vi "SampleListWindow.vi"() -> ()   [LabVIEW 2013]
doc: "The UI for the SampleList that handles the processing of multile samples"
uses:
  Classes/Flags/flag.lvclass
panel:
  out "Analysis Clipboard":string[](array[string])
  out "next sample":u16
  in  "Save button":bool
  in  "load button":bool
  in  "Add sample button":bool
  in  "Add blank button":bool
  out "error out":errorcluster
  in  "error in (no error)":errorcluster
  in  "Start/Stop Button":bool
  in  "Delete Button":bool
  in  "Add std button":bool
  in  "SampleList":i32(listbox)
  # "Add to list"
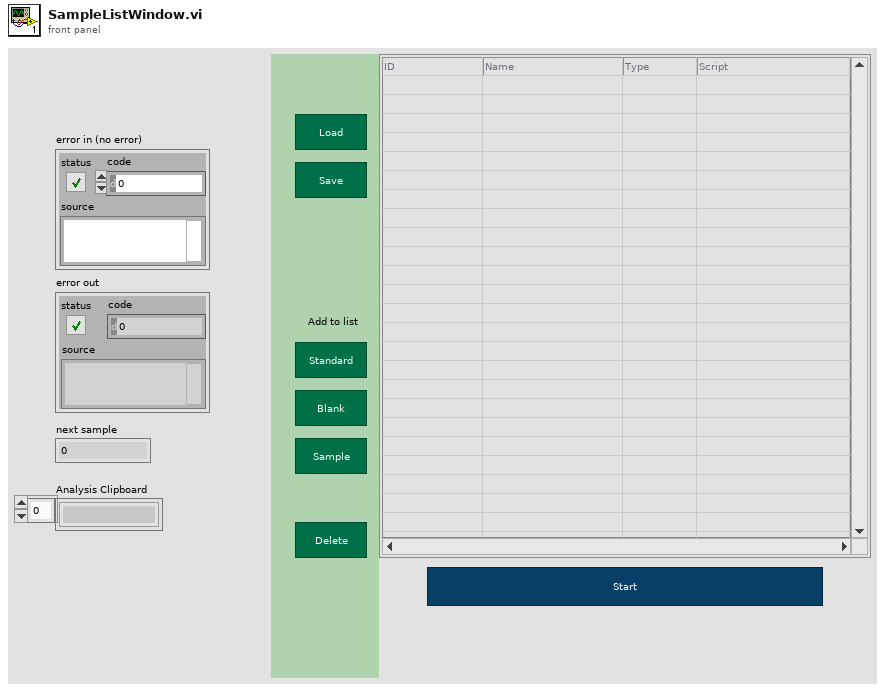
[diagram p1: front panel]
types:
  T1 = typedef "eventvkey.ctl" = enum16{"ASCII", "Enter", "Return", "Shift", "Ctrl", "Alt", "Cmd", "Opt", "Caps", "NumLock", "Clear", "Break", "Up", "Down", "Left", "Right", "Insert", "Delete", "Home", "End", "PageUp", "PageDown", "Escape", "Help", "Pause", "ScrollLock", "F1", "F2", "F3", "F4", "F5", "F6", "F7", "F8", "F9", "F10", "F11", "F12", "F13", "F14", "F15", "F16", "F17", "F18", "F19", "F20", "F21", "F22", "F23", "F24", "Play", "VolumeUp", "VolumeDown", "Mute", "Two Byte Char"}
  T2 = cluster{"Shift":bool, "Ctrl":bool, "Alt":bool, "Cmd":bool, "Opt":bool}
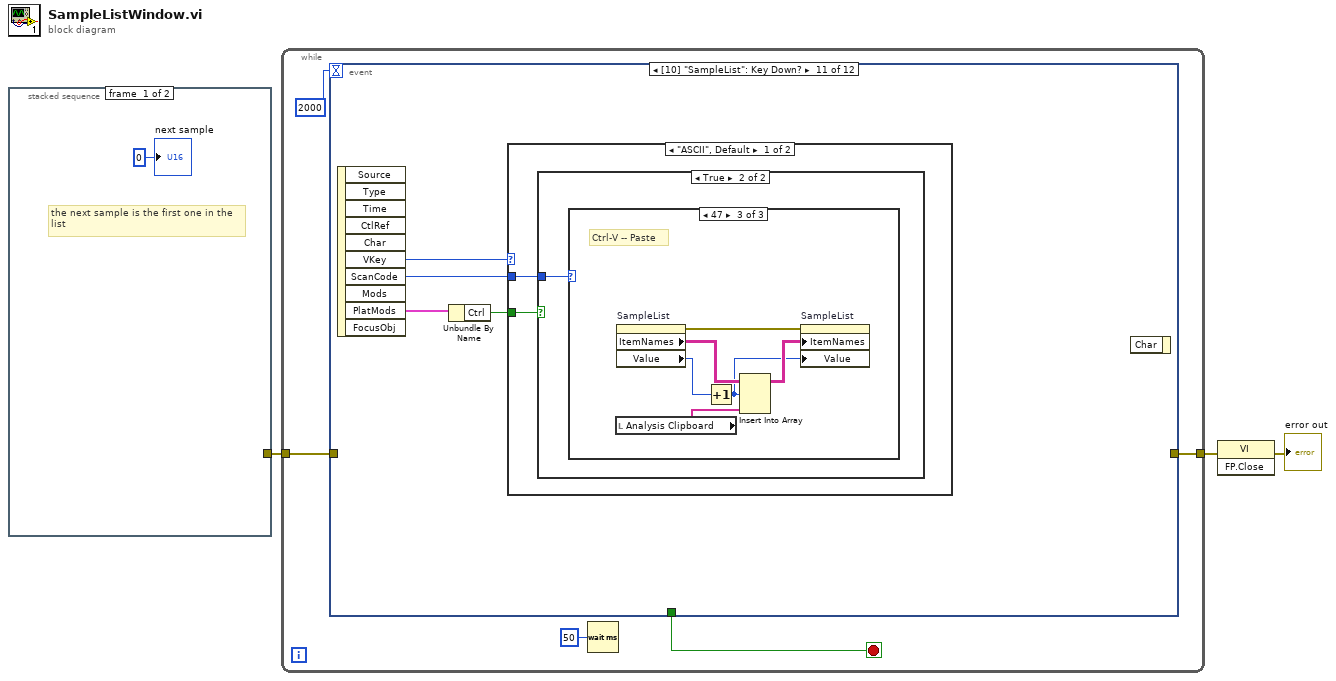
[diagram p0: block diagram]
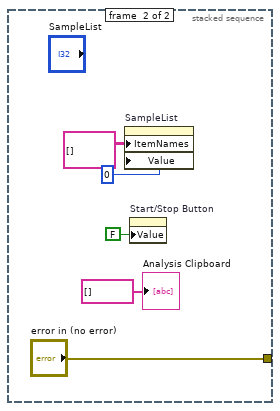
[diagram p2: hidden frame]
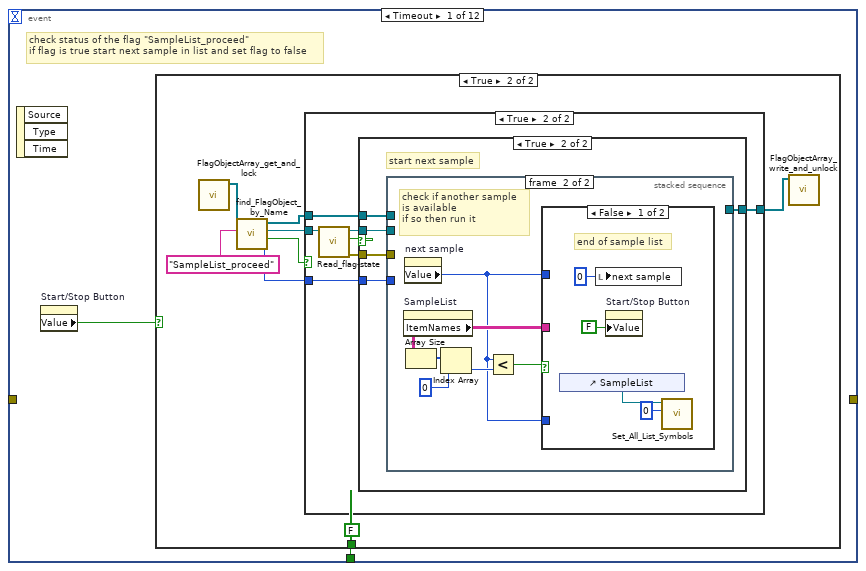
[diagram p3: hidden frame]
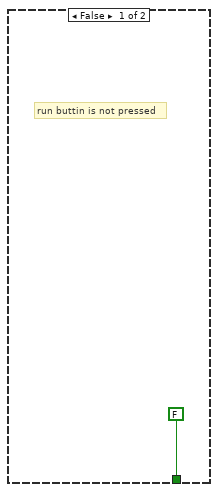
[diagram p4: hidden frame]
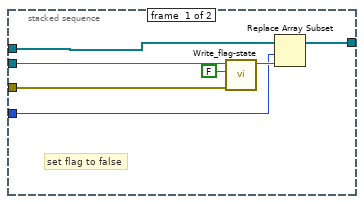
[diagram p7: hidden frame]
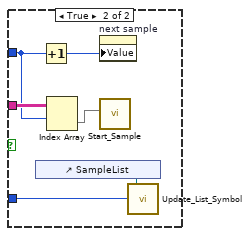
[diagram p8: hidden frame]
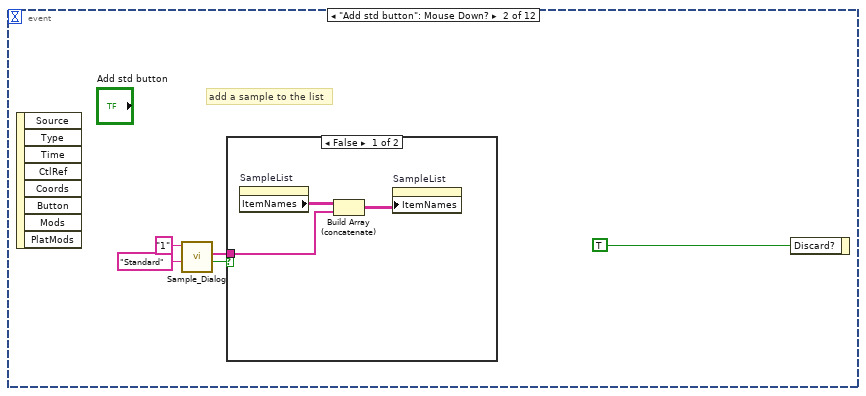
[diagram p9: hidden frame]
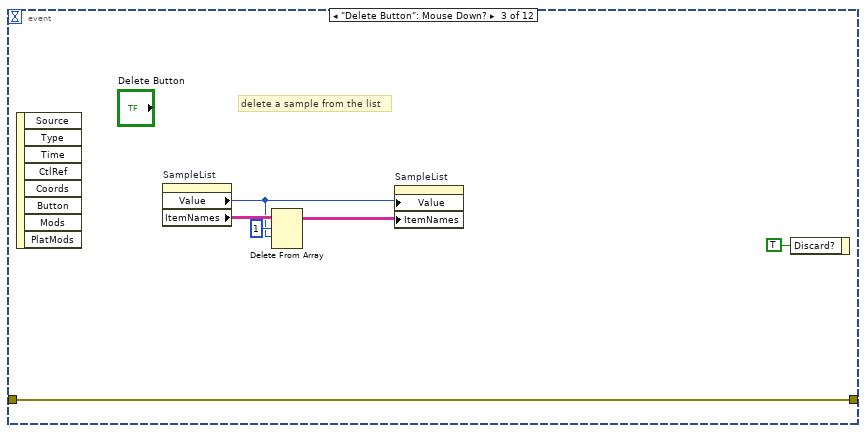
[diagram p11: hidden frame]
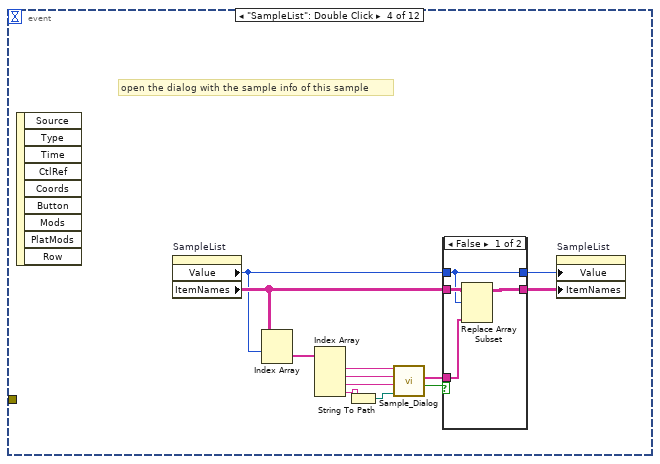
[diagram p12: hidden frame]
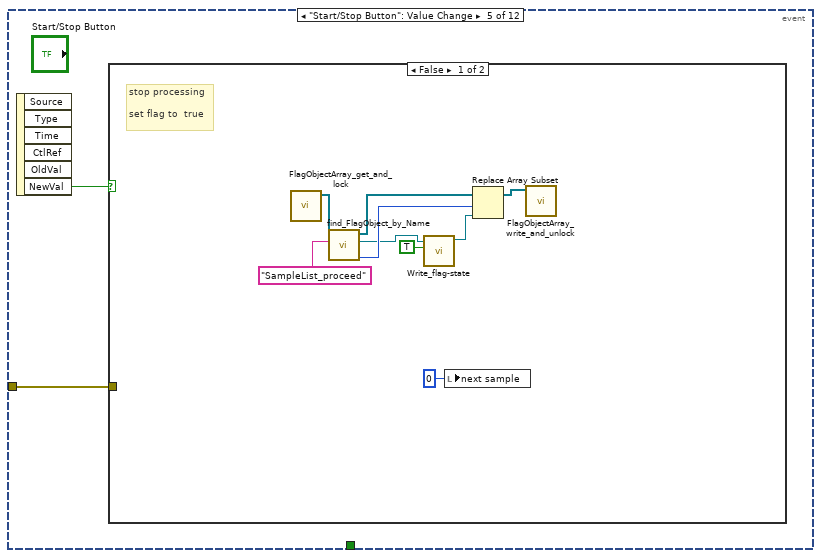
[diagram p14: hidden frame]
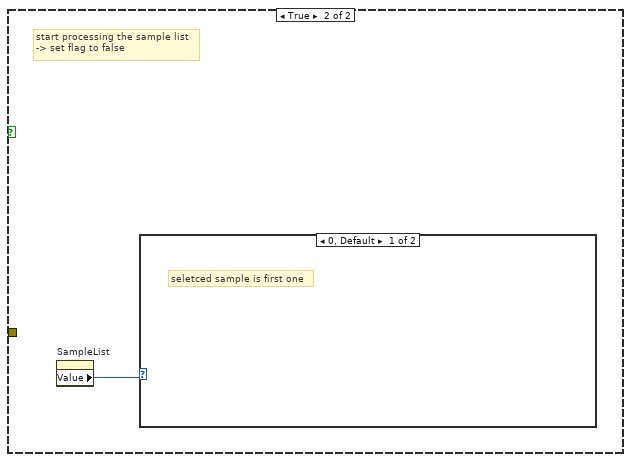
[diagram p15: hidden frame]
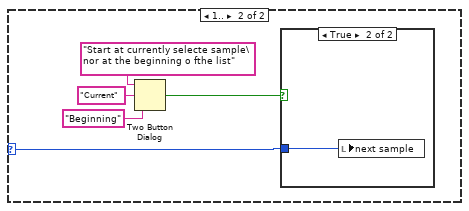
[diagram p16: hidden frame]
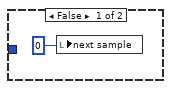
[diagram p17: hidden frame]
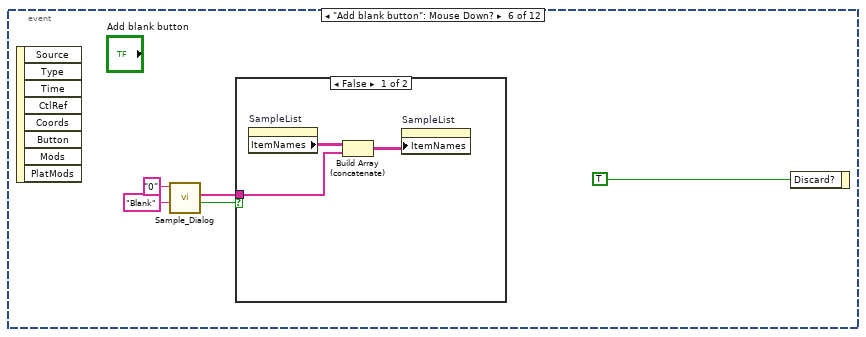
[diagram p18: hidden frame]
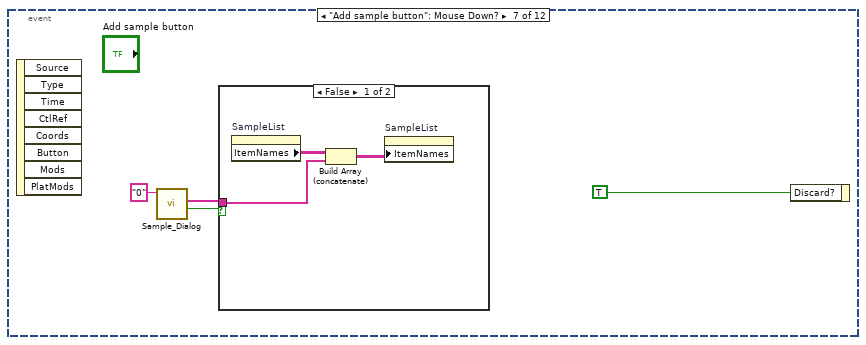
[diagram p20: hidden frame]
diagram:
  n1 = stacked-sequence {
    tunnel: [_ "error in (no error)"] -> w3
    frame #0 {
      # "the next sample is the first one in the\nlist"
      "next sample" <- u16 0 ("current sample")
    }
    frame #1 {
      n2 = property on="SampleList" class="MCListbox (strict)"("ItemNames"=string[][] [] ("Item Names"), "Value"=0 ("SampleList")) -> ()  [unwired: 2 in, 2 out]
      n3 = property on="Start/Stop Button" class="Bool (strict)"("Value"=FALSE ("Start/Stop Button")) -> ()  [unwired: 2 in, 2 out]
      "Analysis Clipboard" <- string[] [] ("Analysis Clipboard")
    }
  }
  n4 = while {
    tunnel: w3 -> [w12]
    tunnel: [w11] -> w2
    stop <- w14 stop-if-true
    n5 = event shown="[10] \"SampleList\": Key Down?" {
      selector: _ -> [_ _ _ _ _ _ _ _ _ _ _ _]
      dyn-events: _ -> [_ _ _ _ _ _ _ _ _ _ _ _]
      timeout: 2000 -> [_ _ _ _ _ _ _ _ _ _ _ _]
      tunnel: [w16 _ _ _ _ _ _ _ _ _ _ w193] -> w14
      tunnel: w12 -> [_ _ w76 _ w96 _ _ _ _ _ _ w191]
      tunnel: [_ _ w76 _ _ _ _ _ _ _ _ w191] -> w11
      event Timeout {
        # "check status of the flag \"SampleList_proceed\"\nif flag is true start next sample in list and set flag to false"
        n6 = event-data() -> ()  [unwired: 1 in, 3 out]
        n7 = property on="Start/Stop Button" class="Bool (strict)"() -> ("Value"=w15:bool)  [unwired: 2 in, 2 out]
        n8 = case shown="True" w15 {
          tunnel: [FALSE FALSE] -> w16
          frame False {
            # "run buttin is not pressed"
          }
          frame True {
            n9 = call "FlagObjectArray_get_and_lock.vi"() -> ("FlagObjects"=w24:refnum<class "flag.lvclass">[])  [unwired: 10 in, 1 out]
            n10 = call "find_FlagObject_by_Name.vi"("Flag Name"="SampleList_proceed", "FlagObj Array"=w24) -> ("index of Object in Array"=w18:i32, "found?"=w21:bool, "found FlagObj out"=w22:refnum<class "flag.lvclass">, "FlagObj Array out"=w20:refnum<class "flag.lvclass">[])  [unwired: 6 in]
            n11 = case shown="True" w21 {
              tunnel: w22 -> [_ w33]
              tunnel: w20 -> [w26 w31]
              tunnel: [w26 w29] -> w19
              tunnel: w18 -> [_ w27]
              frame False {
              }
              frame True {
                n12 = call-dynamic "Read_flag-state.vi"("flag in"=w33) -> ("error out"=w28:errorcluster, "flag state"=w30:bool, "flag out"=w32:refnum<class "flag.lvclass">)  [unwired: 8 in]
                n13 = case shown="True" w30 {
                  tunnel: w32 -> [_ w39]
                  tunnel: w31 -> [w34 w37]
                  tunnel: [w34 w35] -> w29
                  tunnel: w28 -> [_ w38]
                  tunnel: w27 -> [_ w36]
                  frame False {
                    # "do nothing, flag is still false"
                  }
                  frame True {
                    # "start next sample"
                    n14 = stacked-sequence {
                      tunnel: w39 -> [w46 _]
                      tunnel: w38 -> [w45 _]
                      tunnel: w37 -> [w43 _]
                      tunnel: w36 -> [w41 _]
                      tunnel: [w40 _] -> w35
                      frame #0 {
                        # "set flag to false"
                        n15 = call-dynamic "Write_flag-state.vi"("error in (no error)"=w45, "flag state"=FALSE, "flag in"=w46) -> ("flag out"=w42:refnum<class "flag.lvclass">)  [unwired: 7 in, 1 out]
                        n16 = Replace Array Subset(array=w43, new element=w42, index=w41) -> (w40:refnum<class "flag.lvclass">[])
                      }
                      frame #1 {
                        # "check if another sample\nis available\nif so then run it"
                        n17 = property on="SampleList" class="MCListbox (strict)"() -> ("ItemNames"=w52:string[][])  [unwired: 2 in, 2 out]
                        n18 = property on="next sample" class="DigNum (strict)"() -> ("Value"=w47:u16)  [unwired: 2 in, 2 out]
                        n19 = Array Size(array=w52) -> (size(s)=w51:i32[])
                        n20 = Index Array(array=w51, index=0) -> (element=w49:i32)
                        n21 = Less?(x=w47, y=w49) -> (x < y?=w48:bool)
                        n22 = case shown="False" w48 {
                          tunnel: w52 -> [_ w60]
                          tunnel: w47 -> [_ w59]
                          tunnel: w47 -> [_ w57]
                          frame False {
                            # "end of sample list"
                            n23 = control-ref of="SampleList"() -> (w54:refnum<vi>)
                            n24 = local write "next sample"(u16 0 ("next sample")) -> ()
                            n25 = property on="Start/Stop Button" class="Bool (strict)"("Value"=FALSE ("Start/Stop Button")) -> ()  [unwired: 2 in, 2 out]
                            n26 = call "Set_All_List_Symbols.vi"("symbol value"=u16 0, "MulticolumnListbox in"=w54) -> ()  [unwired: 10 in]
                          }
                          frame True {
                            n27 = control-ref of="SampleList"() -> (w58:refnum<vi>)
                            n28 = Increment(x=w59) -> (x+1=w61:u16)
                            n29 = Index Array(array=w60, index (row)=w59) -> (element=w62:string[])  [unwired: 1 in]
                            n30 = property on="next sample" class="DigNum (strict)"("Value"=w61) -> ()  [unwired: 2 in, 2 out]
                            n31 = call "Start_Sample.vi"("SampleList Data"=w62) -> ()  [unwired: 10 in, 1 out]
                            n32 = call "Update_List_Symbol.vi"("current sample"=w57, "MulticolumnListbox in"=w58) -> ()  [unwired: 10 in]
                          }
                        }
                      }
                    }
                  }
                }
              }
            }
            n33 = call "FlagObjectArray_write_and_unlock.vi"("FlagObjects"=w19) -> ()  [unwired: 10 in, 1 out]
          }
        }
      }
      event "Add std button": Mouse Down? {
        # "add a sample to the list"
        n34 = event-data() -> ()  [unwired: 1 in, 8 out]
        n35 = call "Sample_Dialog.vi"("Type"="Standard", "ID"="1") -> ("Canceled?"=w63:bool, "AnalysisData Out"=w64:string[])  [unwired: 8 in]
        n36 = case shown="False" w63 {
          tunnel: w64 -> [w68 _]
          frame False {
            n37 = property on="SampleList" class="MCListbox (strict)"() -> ("ItemNames"=w70:string[][])  [unwired: 2 in, 2 out]
            n38 = Build Array (concatenate)(w70, w68) -> (w69:string[][])
            n39 = property on="SampleList" class="MCListbox (strict)"("ItemNames"=w69) -> ()  [unwired: 2 in, 2 out]
          }
          frame True {
          }
        }
        n40 = event-data("Discard?"=TRUE) -> ()  [unwired: 1 in, 1 out]
      }
      event "Delete Button": Mouse Down? {
        # "delete a sample from the list"
        n41 = event-data() -> ()  [unwired: 1 in, 8 out]
        n42 = property on="SampleList" class="MCListbox (strict)"() -> ("Value"=w73:i32, "ItemNames"=w75:string[][])  [unwired: 2 in, 2 out]
        n43 = Delete From Array(array=w75, length=1, index (row)=w73) -> (array with subset deleted=w72:string[][])  [unwired: 1 in, 1 out]
        n44 = property on="SampleList" class="MCListbox (strict)"("Value"=w73, "ItemNames"=w72) -> ()  [unwired: 2 in, 2 out]
        n45 = event-data("Discard?"=TRUE) -> ()  [unwired: 1 in, 1 out]
      }
      event "SampleList": Double Click {
        # "open the dialog with the sample info of this sample"
        n46 = event-data() -> ()  [unwired: 1 in, 9 out]
        n47 = property on="SampleList" class="MCListbox (strict)"() -> ("Value"=w80:i32, "ItemNames"=w81:string[][])  [unwired: 2 in, 2 out]
        n48 = Index Array(array=w81, index (row)=w80) -> (element=w88:string[])  [unwired: 1 in]
        n49 = Index Array(array=w88) -> (element #1=w87:string, element #2=w86:string, element #3=w85:string, element #4=w84:string)  [unwired: 4 in]
        n50 = String To Path(string=w84) -> (path=w83:path)
        n51 = call "Sample_Dialog.vi"("Script"=w83, "Type"=w85, "Name"=w86, "ID"=w87) -> ("Canceled?"=w78:bool, "AnalysisData Out"=w79:string[])  [unwired: 6 in]
        n52 = case shown="False" w78 {
          tunnel: [w92 w94] -> w82
          tunnel: w81 -> [w91 w94]
          tunnel: w80 -> [w89 w93]
          tunnel: w79 -> [w90 _]
          tunnel: [w89 w93] -> w77
          frame False {
            n53 = Replace Array Subset(array=w91, new element=w90, index (row)=w89) -> (w92:string[][])  [unwired: 1 in]
          }
          frame True {
          }
        }
        n54 = property on="SampleList" class="MCListbox (strict)"("Value"=w77, "ItemNames"=w82) -> ()  [unwired: 2 in, 2 out]
      }
      event "Start/Stop Button": Value Change {
        n55 = event-data() -> ("NewVal"=w95:bool)  [unwired: 1 in, 5 out]
        n56 = case shown="False" w95 {
          tunnel: w96 -> [_ _]
          frame False {
            # "stop processing\n\nset flag to  true"
            n57 = call "FlagObjectArray_get_and_lock.vi"() -> ("FlagObjects"=w105:refnum<class "flag.lvclass">[])  [unwired: 10 in, 1 out]
            n58 = call "find_FlagObject_by_Name.vi"("Flag Name"="SampleList_proceed", "FlagObj Array"=w105) -> ("index of Object in Array"=w99:i32, "found FlagObj out"=w98:refnum<class "flag.lvclass">, "FlagObj Array out"=w100:refnum<class "flag.lvclass">[])  [unwired: 6 in, 1 out]
            n59 = call-dynamic "Write_flag-state.vi"("flag state"=TRUE, "flag in"=w98) -> ("flag out"=w102:refnum<class "flag.lvclass">)  [unwired: 8 in, 1 out]
            n60 = local write "next sample"(u16 0 ("next sample")) -> ()
            n61 = Replace Array Subset(array=w100, new element=w102, index=w99) -> (w101:refnum<class "flag.lvclass">[])
            n62 = call "FlagObjectArray_write_and_unlock.vi"("FlagObjects"=w101) -> ()  [unwired: 10 in, 1 out]
          }
          frame True {
            # "start processing the sample list\n-> set flag to false"
            n63 = property on="SampleList" class="MCListbox (strict)"() -> ("Value"=w106:i32)  [unwired: 2 in, 2 out]
            n64 = case shown="0, Default" w106 {
              selector: w106 -> [_ w107]
              frame 0, Default {
                # "seletced sample is first one"
              }
              frame 1.. {
                n65 = Two Button Dialog(message="Start at currently selecte sample\nor at the beginning o fthe list", 1:"Beginning" ("F button name (\"Cancel\")"), 2:"Current" ("T button name (\"OK\")")) -> (T button?=w108:bool)
                n66 = case shown="True" w108 {
                  tunnel: w107 -> [_ w113]
                  frame False {
                    n67 = local write "next sample"(0 ("SampleList")) -> ()
                  }
                  frame True {
                    n68 = local write "next sample"(w113) -> ()
                  }
                }
              }
            }
          }
        }
      }
      event "Add blank button": Mouse Down? {
        n69 = event-data() -> ()  [unwired: 1 in, 8 out]
        n70 = call "Sample_Dialog.vi"("Type"="Blank", "ID"="0") -> ("Canceled?"=w114:bool, "AnalysisData Out"=w115:string[])  [unwired: 8 in]
        n71 = case shown="False" w114 {
          tunnel: w115 -> [w119 _]
          frame False {
            n72 = property on="SampleList" class="MCListbox (strict)"() -> ("ItemNames"=w121:string[][])  [unwired: 2 in, 2 out]
            n73 = Build Array (concatenate)(w121, w119) -> (w120:string[][])
            n74 = property on="SampleList" class="MCListbox (strict)"("ItemNames"=w120) -> ()  [unwired: 2 in, 2 out]
          }
          frame True {
          }
        }
        n75 = event-data("Discard?"=TRUE) -> ()  [unwired: 1 in, 1 out]
      }
      event "Add sample button": Mouse Down? {
        n76 = event-data() -> ()  [unwired: 1 in, 8 out]
        n77 = call "Sample_Dialog.vi"("ID"="0") -> ("Canceled?"=w122:bool, "AnalysisData Out"=w123:string[])  [unwired: 9 in]
        n78 = case shown="False" w122 {
          tunnel: w123 -> [w126 _]
          frame False {
            n79 = property on="SampleList" class="MCListbox (strict)"() -> ("ItemNames"=w128:string[][])  [unwired: 2 in, 2 out]
            n80 = Build Array (concatenate)(w128, w126) -> (w127:string[][])
            n81 = property on="SampleList" class="MCListbox (strict)"("ItemNames"=w127) -> ()  [unwired: 2 in, 2 out]
          }
          frame True {
          }
        }
        n82 = event-data("Discard?"=TRUE) -> ()  [unwired: 1 in, 1 out]
      }
      event "load button": Mouse Down? {
        n83 = event-data() -> ()  [unwired: 1 in, 8 out]
        n84 = Current VI's Path() -> (path=w135:path)
        n85 = call "current_vi_path_stripped2.vi"("current VI Path"=w135) -> ("current VI Path stripped out"=w130:path)  [unwired: 3 in, 1 out]
        n86 = Strip Path(path=w130) -> (stripped path=w129:path)  [unwired: 1 out]
        n87 = Build Path(base path=w129, name or relative path="SampleLists") -> (appended path=w134:path)
        n88 = call "File Dialog2"("start path"=w134) -> ("selected path"=w132:path, "cancelled"=w133:bool, "error out"=w131:errorcluster)  [unwired: 11 in, 1 out]
        n89 = case shown="False" w133 {
          tunnel: w132 -> [w139 _]
          tunnel: w131 -> [_ _]
          frame False {
            n90 = Read from Text File(file (use dialog)=w139) -> (refnum out=w146:refnum<file>, text=w144:string, error out=w145:errorcluster)  [unwired: 3 in, 1 out]
            n91 = Spreadsheet String To Array(delimiter (Tab)=";", format string="%s", spreadsheet string=w144, array type (2D Dbl)=string[][] []) -> (array=w140:string[][])
            n92 = Close File(refnum=w146, error in=w145) -> ()  [unwired: 2 out]
            n93 = property on="SampleList" class="MCListbox (strict)"("ItemNames"=w140, "Value"=0 ("SampleList")) -> ()  [unwired: 2 in, 2 out]
          }
          frame True {
          }
        }
        n94 = event-data("Discard?"=TRUE) -> ()  [unwired: 1 in, 1 out]
      }
      event "Save button": Mouse Down? {
        # "save data to a text file"
        n95 = event-data() -> ()  [unwired: 1 in, 8 out]
        n96 = Current VI's Path() -> (path=w153:path)
        n97 = call "current_vi_path_stripped2.vi"("current VI Path"=w153) -> ("current VI Path stripped out"=w148:path)  [unwired: 3 in, 1 out]
        n98 = Strip Path(path=w148) -> (stripped path=w147:path)  [unwired: 1 out]
        n99 = property on="SampleList" class="MCListbox (strict)"() -> ("ItemNames"=w156:string[][])  [unwired: 2 in, 2 out]
        n100 = Build Path(base path=w147, name or relative path="SampleLists") -> (appended path=w152:path)
        n101 = call "File Dialog"("start path"=w152) -> ("selected path"=w150:path, "cancelled"=w151:bool, "error out"=w149:errorcluster)  [unwired: 11 in, 1 out]
        n102 = Array To Spreadsheet String(delimiter (Tab)=";", array=w156, 3:"%s" ("format string")) -> (spreadsheet string=w155:string)
        n103 = case shown="False" w151 {
          tunnel: w155 -> [w163 _]
          tunnel: w150 -> [w160 _]
          tunnel: w149 -> [_ _]
          frame False {
            n104 = Write to Text File(file (use dialog)=w160, text=w163) -> (refnum out=w162:refnum<file>, error out=w161:errorcluster)  [unwired: 2 in, 1 out]
            n105 = Close File(refnum=w162, error in=w161) -> ()  [unwired: 2 out]
          }
          frame True {
          }
        }
        n106 = event-data("Discard?"=TRUE) -> ()  [unwired: 1 in, 1 out]
      }
      event "SampleList": Shortcut Menu Selection? (App) {
        n107 = event-data() -> ("ItemTag"=w165:string)  [unwired: 1 in, 7 out]
        n108 = case shown="\"APP_SC_COPY_DATA\"" w165 {
          frame "False", Default {
          }
          frame "APP_SC_COPY_DATA" {
            # "copy the data of the currently selected line"
            # "copy data"
            n109 = property on="SampleList" class="MCListbox (strict)"() -> ("ItemNames"=w168:string[][], "Value"=w167:i32)  [unwired: 2 in, 2 out]
            n110 = Index Array(array=w168, index (row)=w167) -> (element=w166:string[])  [unwired: 1 in]
            n111 = local write "Analysis Clipboard"(w166) -> ()
          }
          frame "APP_SC_PASTE_DATA" {
            # "paste the data after the currently selected line"
            # "paste data"
            n112 = local read "Analysis Clipboard"() -> (w172:string[])
            n113 = property on="SampleList" class="MCListbox (strict)"() -> (error out=w170:errorcluster, "ItemNames"=w174:string[][], "Value"=w173:i32)  [unwired: 2 in, 1 out]
            n114 = Increment(x=w173) -> (x+1=w169:i32)
            n115 = Insert Into Array(array=w174, index (row)=w169, new element=w172) -> (w171:string[][])  [unwired: 1 in]
            n116 = property on="SampleList" class="MCListbox (strict)"(error in=w170, "ItemNames"=w171, "Value"=w169) -> ()  [unwired: 1 in, 2 out]
          }
        }
        n117 = event-data("Discard?"=TRUE) -> ()  [unwired: 1 in, 1 out]
      }
      event "SampleList": Key Down? {
        n118 = event-data() -> ("VKey"=w176:T1, "ScanCode"=w175:i16, "PlatMods"=w178:T2)  [unwired: 1 in, 7 out]
        n119 = Unbundle By Name(w178) -> ("Ctrl"=w177:bool)
        n120 = case shown="\"ASCII\", Default" w176 {
          tunnel: w177 -> [w180 _]
          tunnel: w175 -> [w179 _]
          frame "ASCII", Default {
            n121 = case shown="True" w180 {
              tunnel: w179 -> [_ w181]
              frame False {
              }
              frame True {
                n122 = case shown="47" w181 {
                  frame 0, Default {
                  }
                  frame 46 {
                    # "Ctrl-C -- Copy"
                    n123 = property on="SampleList" class="MCListbox (strict)"() -> ("ItemNames"=w184:string[][], "Value"=w183:i32)  [unwired: 2 in, 2 out]
                    n124 = Index Array(array=w184, index (row)=w183) -> (element=w182:string[])  [unwired: 1 in]
                    n125 = local write "Analysis Clipboard"(w182) -> ()
                  }
                  frame 47 {
                    # "Ctrl-V -- Paste"
                    n126 = local read "Analysis Clipboard"() -> (w188:string[])
                    n127 = property on="SampleList" class="MCListbox (strict)"() -> (error out=w186:errorcluster, "ItemNames"=w190:string[][], "Value"=w189:i32)  [unwired: 2 in, 1 out]
                    n128 = Increment(x=w189) -> (x+1=w185:i32)
                    n129 = Insert Into Array(array=w190, index (row)=w185, new element=w188) -> (w187:string[][])  [unwired: 1 in]
                    n130 = property on="SampleList" class="MCListbox (strict)"(error in=w186, "ItemNames"=w187, "Value"=w185) -> ()  [unwired: 1 in, 2 out]
                  }
                }
              }
            }
          }
          frame "Enter" {
          }
        }
        n131 = event-data() -> ()  [unwired: 2 in, 1 out]
      }
      event Panel Close? {
        # "close the vi"
        n132 = event-data() -> ()  [unwired: 1 in, 4 out]
        n133 = Two Button Dialog(message="Do you really want to close?") -> (T button?=w193:bool)  [unwired: 2 in]
        n134 = event-data("Discard?"=TRUE) -> ()  [unwired: 1 in, 1 out]
      }
    }
    n135 = Wait (ms)(milliseconds to wait=u32 50) -> ()  [unwired: 1 out]
  }
  n136 = invoke class="VI" method="FP.Close"(error in=w2) -> (error out=→"error out":errorcluster)  [unwired: 2 in, 2 out]
